vi "rs3_close all2.vi"(4 "Stop and Exit":bool, 6 "rscontext":u64, 7 "queue in":u64, 8 "error in (no error)":errorcluster, 9 "device_list":u64, 10 "Dev in":u64, 11 "Sensor in":u64) -> (0 "error out (no error)":errorcluster, 3 "Close Error":string)   [LabVIEW 2017, in "libRealSense3.lvlib"]
doc: "It is important to close everything properly at the end. Use this VI to clean up and close the RealSense device, queue, sensor, and device list."
uses:
  libRealSense3.lvlib
panel:
  # "RS3 Close All"
  # "(C) Intel Corp. 2017,  AGJ"
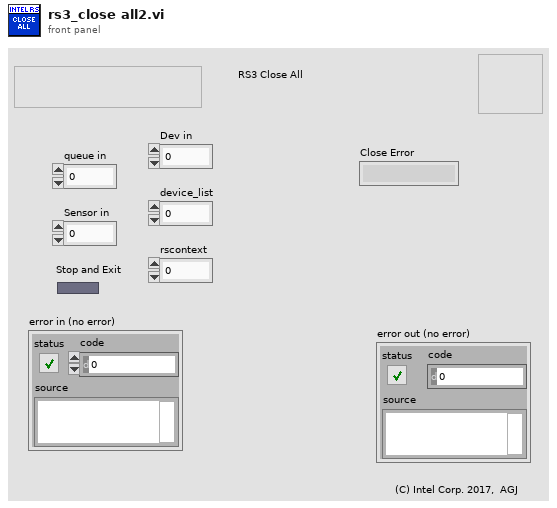
[diagram p1: front panel]
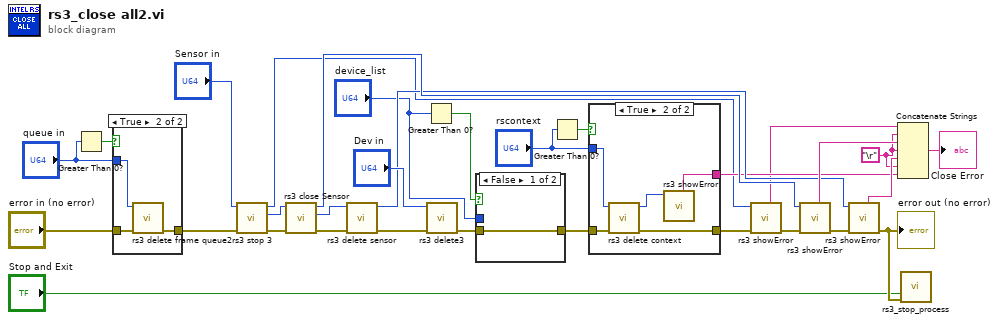
[diagram p0: block diagram]
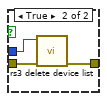
[diagram p2: hidden frame]
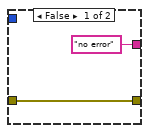
[diagram p4: hidden frame]
diagram:
  w14 = "\r"
  n1 = Greater Than 0?(x="queue in") -> (x > 0?=w10:bool)
  n2 = case shown="True" w10 {
    tunnel: "error in (no error)" -> [w32 w35]
    tunnel: "queue in" -> [_ w34]
    tunnel: [w32 w33] -> w18
    frame False {
    }
    frame True {
      n3 = call "rs3 delete frame queue2.vi"("error in (no error)"=w35, "queue"=w34) -> ("error out"=w33:errorcluster)  [unwired: 9 in]
    }
  }
  n4 = call "rs3 stop 3.vi"("error in (no error)"=w18, "sensor"="Sensor in") -> ("error out"=w17:errorcluster, "sensor out"=w15:u64, "error"=w12:u64)  [unwired: 7 in]
  n5 = call "rs3 close Sensor.vi"("error in (no error)"=w17, "sensor"=w15) -> ("error out"=w29:errorcluster, "device out"=w28:u64, "error"=w21:u64)  [unwired: 7 in]
  n6 = call "rs3 delete sensor.vi"("error in (no error)"=w29, "sensor"=w28) -> ("error out"=w30:errorcluster, "error"=w20:u64)  [unwired: 8 in]
  n7 = Greater Than 0?(x="device_list") -> (x > 0?=w3:bool)
  n8 = call "rs3 delete3.vi"("error in (no error)"=w30, "device"="Dev in") -> ("error out"=w25:errorcluster)  [unwired: 9 in]
  n9 = case shown="False" w3 {
    tunnel: [w36 w39] -> w27
    tunnel: w25 -> [w36 w38]
    tunnel: "device_list" -> [_ w37]
    frame False {
    }
    frame True {
      n10 = call "rs3 delete device list.vi"("error in (no error)"=w38, "device list"=w37) -> ("error out"=w39:errorcluster)  [unwired: 9 in]
    }
  }
  n11 = Greater Than 0?(x="rscontext") -> (x > 0?=w8:bool)
  n12 = case shown="True" w8 {
    tunnel: w27 -> [w40 w46]
    tunnel: [w40 w45] -> w7
    tunnel: ["no error" ("Error summary") w43] -> w19
    tunnel: "rscontext" -> [_ w42]
    frame False {
    }
    frame True {
      n13 = call "rs3 delete context.vi"("error in (no error)"=w46, "context"=w42) -> ("error out"=w45:errorcluster, "error"=w44:u64)  [unwired: 8 in]
      n14 = call "rs3 showError.vi"("error"=w44) -> ("Error summary"=w43:string)  [unwired: 6 in, 4 out]
    }
  }
  n15 = call "rs3 showError.vi"("error in (no error)"=w7, "error"=w12) -> ("error out"=w6:errorcluster, "Error summary"=w13:string)  [unwired: 5 in, 3 out]
  n16 = call "rs3 showError.vi"("error in (no error)"=w6, "error"=w21) -> ("error out"=w5:errorcluster, "Error summary"=w24:string)  [unwired: 5 in, 3 out]
  n17 = call "rs3 showError.vi"("error in (no error)"=w5, "error"=w20) -> ("error out"=w2:errorcluster, "Error summary"=w23:string)  [unwired: 5 in, 3 out]
  "error out (no error)" <- w2
  n18 = Concatenate Strings(w13, w14, w24, w14, w23, w14, w19) -> (→"Close Error":string)
  n19 = call "rs3_stop_process.vi"("STOP and EXIT"="Stop and Exit", "error in (no error)"=w2) -> ()  [unwired: 14 in]
